vi "Map UUID List Error Check.vi"(1 "indices":i32[](array[numeric])=[-1, 1, 3, 4, -1], 2 "UUIDs":string[](array[string])=["A", "B", "C", "D", "E"]) -> (0 "error constant":errorcluster)   [LabVIEW 2020]
uses:
  Match 1D Array Elements/Match 1D Array Elements - double.vi
  Index Array Elements/Index Array Elements - string.vi
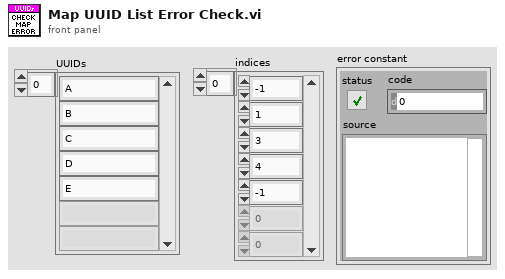
[diagram p1: front panel]
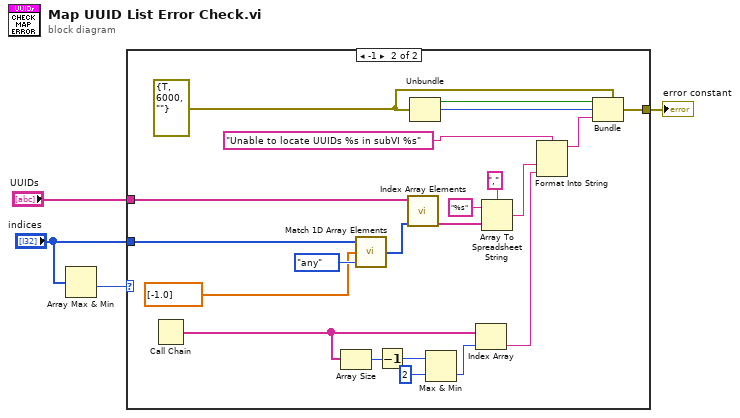
[diagram p0: block diagram]
diagram:
  n1 = Array Max & Min(array="indices") -> (min value=w4:i32)  [unwired: 3 out]
  n2 = case shown="-1" w4 {
    tunnel: "indices" -> [_ w25]
    tunnel: "UUIDs" -> [_ w21]
    tunnel: [_ w11] -> w1
    frame Default {
    }
    frame -1 {
      w9 = errorcluster {"status"=TRUE, "code"=6000, "source"=""} ("error constant")
      n3 = Call Chain() -> (call chain=w17:string[])
      n4 = Array Size(array=w17) -> (size(s)=w15:i32)
      n5 = call-poly "Match 1D Array Elements.vi"("mode (any)"=enum16{"any", "each"}."any", "elements (none)"=dbl[] [-1.0], "1D Array"=w25) -> ("indices"=w22:i32[])
      n6 = Decrement(x=w15) -> (x-1=w10:i32)
      n7 = call-poly "Index Array Elements.vi"("indices (none)"=w22, "1D Array"=w21) -> ("output array"=w20:string[])  [unwired: 5 in]
      n8 = Unbundle(w9) -> ("status"=w13:bool, "code"=w12:i32)  [unwired: 1 out]
      n9 = Max & Min(x=w10, y=2) -> (min(x,y)=w14:i32)  [unwired: 1 out]
      n10 = Index Array(array=w17, index=w14) -> (element=w5:string)
      n11 = Array To Spreadsheet String(delimiter (Tab)=",", array=w20, 3:"%s" ("format string")) -> (spreadsheet string=w6:string)
      n12 = Format Into String(format string="Unable to locate UUIDs %s in subVI %s" ("source"), w6, w5) -> (resulting string=w8:string)  [unwired: 2 in, 1 out]
      n13 = Bundle(cluster=w9, "status"=w13, "code"=w12, "source"=w8) -> (w11:errorcluster)
    }
  }
  "error constant" <- w1
